vi "Teleop.vi"(10 "Match Info":T1={"Autonomous Elapsed Seconds"=0.0, "TeleOp Elapsed Seconds"=0.0, "Disabled Elapsed Seconds"=0.0, "Visited Autonomous"=FALSE, "Visited TeleOp"=FALSE, "Visited Disabled"=FALSE, "Autonomous Settings"={"Autonomous Style"=enum."Independent", "VI Refnum"=refnum}}, 11 "Call Context":T2) -> ()   [LabVIEW 2019]
doc: "This VI is called for each TeleOp packet received from the DS where the robot is not disabled. It is often used to read from the joysticks and update I/O or to update setpoints for timed control loops. It should complete and return within 20 milliseconds or it may miss DS packets."
uses:
  <vilib>/Rock Robotics/WPI/DriverStation/WPI_DriverStationDerivedRobotMode.ctl
  <vilib>/Rock Robotics/WPI/DriverStation/WPI_DriverStationMatch Info.ctl
  <vilib>/Rock Robotics/WPI/ThirdParty/REV Robotics/SPARK MAX/Typedef/Spark MAX Idle Mode.ctl
  Robot Global Data.vi
panel:
  # "Click here to set max"
  # "Click here to set min"
  # "Click here to set max"
  # "Click here to set min"
  # "Click here to set max"
  # "Click here to set min"
  # "Click here to set max"
  # "Click here to set min"
  # "Click here to set max"
  # "Click here to set min"
  # "Click here to set max"
  # "Click here to set min"
  # "Click here to set max"
  # "Click here to set min"
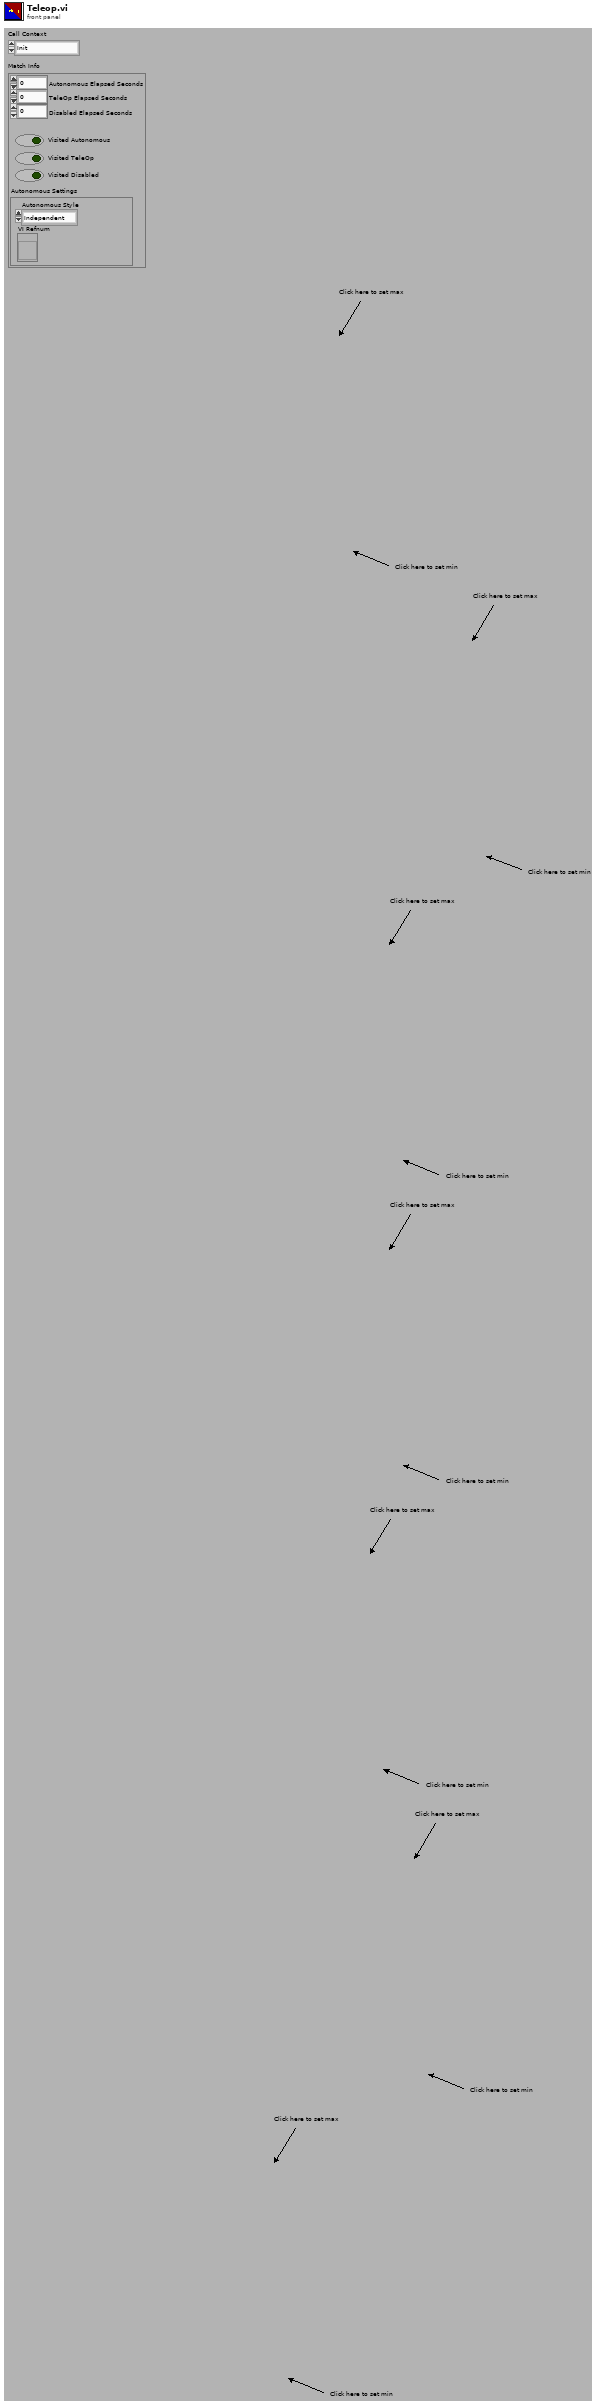
[diagram p1: front panel]
types:
  T1 = typedef "WPI_DriverStationMatch Info.ctl" = cluster{"Autonomous Elapsed Seconds":dbl, "TeleOp Elapsed Seconds":dbl, "Disabled Elapsed Seconds":dbl, "Visited Autonomous":bool, "Visited TeleOp":bool, "Visited Disabled":bool, "Autonomous Settings":cluster{"Autonomous Style":enum16{"Iterative", "Independent"}, "VI Refnum":refnum<vi>}}
  T2 = typedef "WPI_DriverStationDerivedRobotMode.ctl" = enum16{"Init", "Execute", "Stop"}
  T3 = typedef "WPI_MotorControlDeviceRef.ctl" = cluster{"DeviceStatus":errorcluster, "Type":T4, "PWM":cluster{"PWM Channel":T5, "DeadBand":T6}, "CAN":cluster{"Device Number":u8, "SetOutput VI Ref":variant, "GetOutput VI Ref":variant, "Enable VI Ref":variant, "Disable VI Ref":variant, "Data":variant}, "Invert":bool, "DIO PWM":cluster{"PWM \"Enable\" Channel":T5, "DIOChannel":T7, "PWM Rate":dbl}}
  T4 = typedef "WPI_MotorControlType.ctl" = enum16{"PWM", "CAN", "DIO PWM"}
  T5 = typedef "FPGA_DIOPWMChannel.ctl" = enum8{"PWM 0", "PWM 1", "PWM 2", "PWM 3", "PWM 4", "PWM 5", "PWM 6", "PWM 7", "PWM 8", "PWM 9", "PWM MXP 0", "PWM MXP 1", "PWM MXP 2", "PWM MXP 3", "PWM MXP 4", "PWM MXP 5", "PWM MXP 6", "PWM MXP 7", "PWM MXP 8", "PWM MXP 9", "Invalid"}
  T6 = typedef "WPI_PWMDeadband.ctl" = cluster{"Name":string, "maxPositivePwm":i32, "minPositivePwm":i32, "centerPwm":i32, "maxNegativePwm":i32, "minNegativePwm":i32, "angularRange":u16}
  T7 = typedef "FPGA_DIOChannel.ctl" = enum8{"DIO 0", "DIO 1", "DIO 2", "DIO 3", "DIO 4", "DIO 5", "DIO 6", "DIO 7", "DIO 8", "DIO 9", "DIO MXP 0", "DIO MXP 1", "DIO MXP 2", "DIO MXP 3", "DIO MXP 4", "DIO MXP 5", "DIO MXP 6", "DIO MXP 7", "DIO MXP 8", "DIO MXP 9", "DIO MXP 10", "DIO MXP 11", "DIO MXP 12", "DIO MXP 13", "DIO MXP 14", "DIO MXP 15", "SPI Port CS1", "SPI Port CS2", "SPI Port CS3", "SPI Port MISO", "SPI Port MOSI", "Invalid"}
  T8 = typedef "WPI_ServoDeviceRef.ctl" = cluster{"DeviceStatus":errorcluster, "PWM Channel":T5, "DeadBand":T6}
  T9 = typedef "Spark MAX Idle Mode.ctl" = enum16{"Coast", "Brake"}
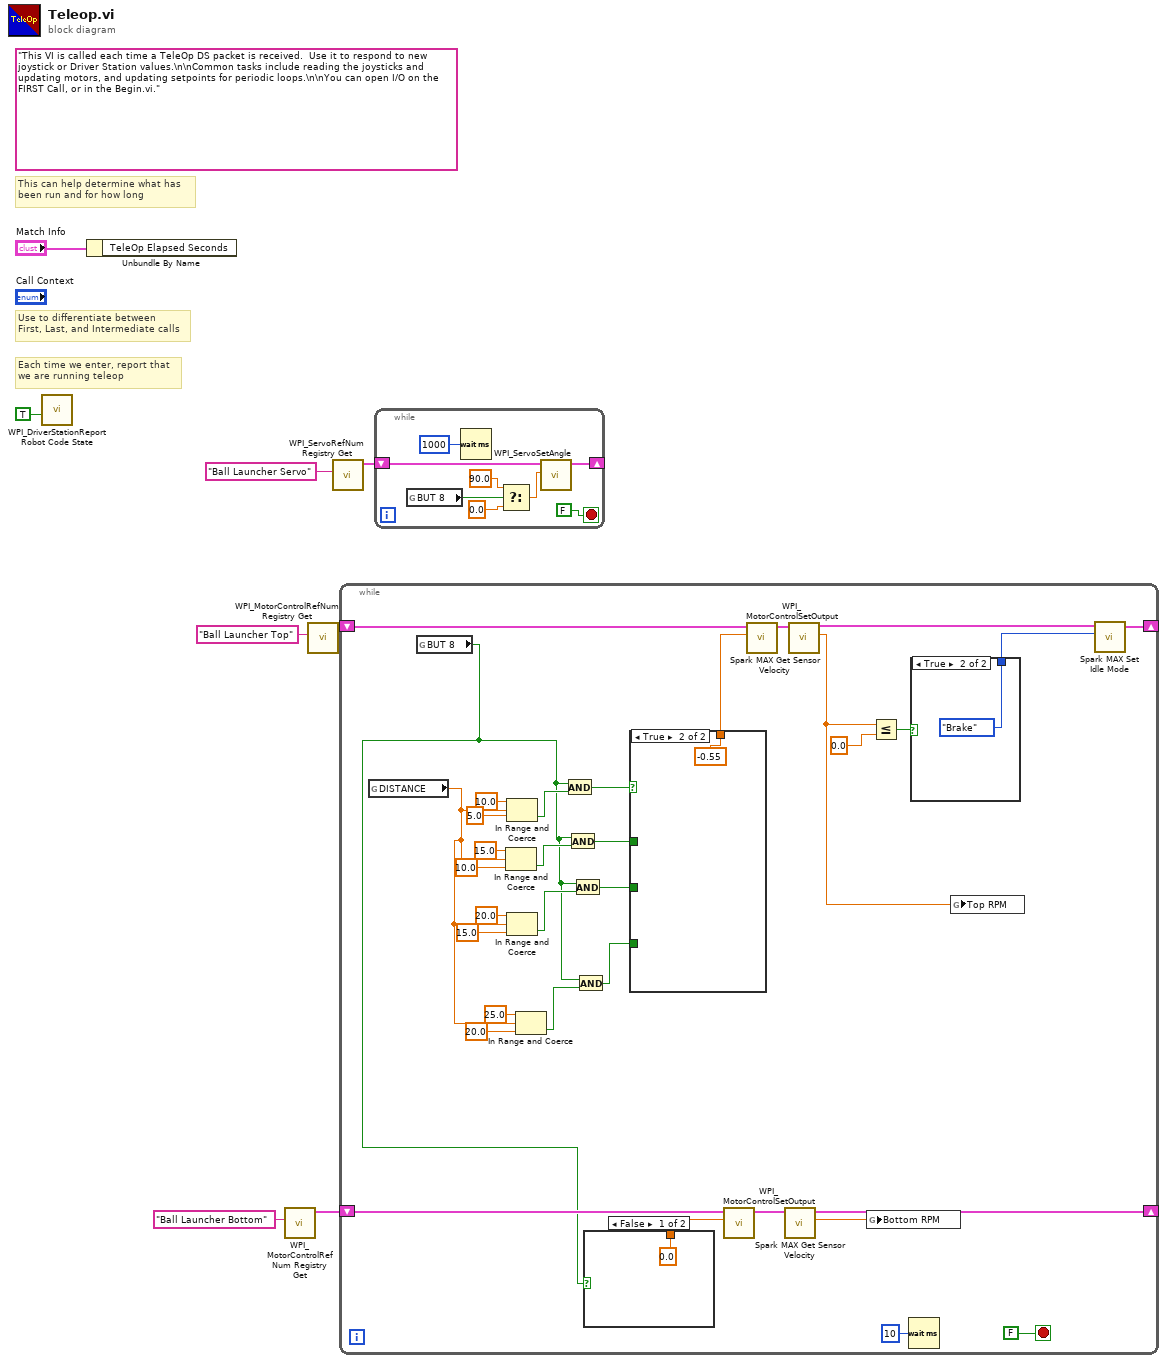
[diagram p0: block diagram]
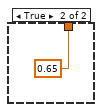
[diagram p2: hidden frame]
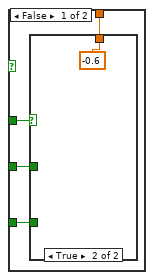
[diagram p3: hidden frame]
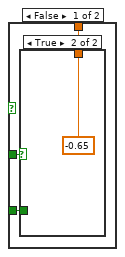
[diagram p4: hidden frame]
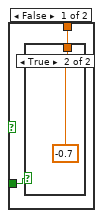
[diagram p5: hidden frame]
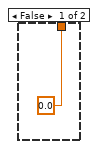
[diagram p6: hidden frame]
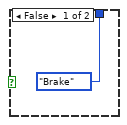
[diagram p7: hidden frame]
diagram:
  (unwired) "This VI is called each time a TeleOp DS packet is received.  Use it to respond to new joystick or Driver Station values.\n\nCommon tasks include reading the joysticks and updating motors, and updating setpoints for periodic loops.\n\nYou can open I/O on the FIRST Call, or in the Begin.vi."
  # "Each time we enter, report that\nwe are running teleop"
  # "Use to differentiate between\nFirst, Last, and Intermediate calls"
  # "This can help determine what has\nbeen run and for how long"
  n1 = call <vilib>:"WPI_DriverStationReport Robot Code State.vi"("TeleOp"=TRUE ("Autonomous")) -> ()  [unwired: 10 in, 1 out]
  n2 = Unbundle By Name("Match Info") -> ()  [unwired: 1 out]
  n3 = call <vilib>:"WPI_MotorControlRefNum Registry Get.vi"("refnum name"="Ball Launcher Bottom") -> ("MotorControlDevRef"=w1:T3)  [unwired: 9 in, 1 out]
  n4 = call <vilib>:"WPI_MotorControlRefNum Registry Get.vi"("refnum name"="Ball Launcher Top") -> ("MotorControlDevRef"=w4:T3)  [unwired: 9 in, 1 out]
  n5 = call <vilib>:"WPI_ServoRefNum Registry Get.vi"("refnum name"="Ball Launcher Servo") -> ("ServoDeviceRef"=w6:T8)  [unwired: 9 in, 1 out]
  n6 = while {
    shift-right: [w37] -> _
    shift-left: w4 -> [w41]
    shift-right: [w32] -> _
    shift-left: w1 -> [w34]
    stop <- FALSE stop-if-true
    n7 = global read "Robot Global Data.vi" "DISTANCE"() -> (w15:dbl)
    n8 = global read "Robot Global Data.vi" "BUT 8"() -> (w10:bool)
    n9 = In Range and Coerce(upper limit=15.0, x=w15, lower limit=10.0) -> (In Range?=w22:bool)  [unwired: 1 out]
    n10 = In Range and Coerce(upper limit=10.0, x=w15, lower limit=5.0) -> (In Range?=w27:bool)  [unwired: 1 out]
    n11 = In Range and Coerce(upper limit=20.0, x=w15, lower limit=15.0) -> (In Range?=w19:bool)  [unwired: 1 out]
    n12 = In Range and Coerce(upper limit=25.0, x=w15, lower limit=20.0) -> (In Range?=w9:bool)  [unwired: 1 out]
    n13 = And(x=w10, y=w27) -> (x .and. y?=w28:bool)
    n14 = And(x=w10, y=w22) -> (x .and. y?=w21:bool)
    n15 = And(x=w10, y=w19) -> (x .and. y?=w20:bool)
    n16 = And(x=w10, y=w9) -> (x .and. y?=w16:bool)
    n17 = case shown="False" w10 {
      tunnel: [0.0 ("Output") 0.65 ("Output")] -> w11
      frame False {
      }
      frame True {
      }
    }
    n18 = case shown="True" w28 {
      tunnel: w21 -> [w48 _]
      tunnel: w20 -> [w47 _]
      tunnel: w16 -> [w46 _]
      tunnel: [w45 -0.55 ("Output")] -> w12
      frame False {
        n19 = case shown="True" w48 {
          tunnel: w47 -> [w51 _]
          tunnel: w46 -> [w50 _]
          tunnel: [w49 -0.6 ("Output")] -> w45
          frame False {
            n20 = case shown="True" w51 {
              tunnel: w50 -> [w53 _]
              tunnel: [w52 -0.65 ("Output")] -> w49
              frame False {
                n21 = case shown="True" w53 {
                  tunnel: [0.0 ("Output") -0.7 ("Output")] -> w52
                  frame False {
                  }
                  frame True {
                  }
                }
              }
              frame True {
              }
            }
          }
          frame True {
          }
        }
      }
      frame True {
      }
    }
    n22 = call <vilib>:"WPI_MotorControlSetOutput.vi"("Output"=w11, "MotorControlDevRef"=w34) -> ("MotorControlDevRef"=w33:T3)  [unwired: 7 in, 2 out]
    n23 = call <vilib>:"WPI_MotorControlSetOutput.vi"("Output"=w12, "MotorControlDevRef"=w41) -> ("MotorControlDevRef"=w42:T3)  [unwired: 7 in, 2 out]
    n24 = call <vilib>:"Spark MAX Get Sensor Velocity.vi"("MotorControlDevRef in"=w33) -> ("Sensor Velocity"=w30:dbl, "MotorControlDevRef out"=w32:T3)  [unwired: 7 in, 2 out]
    n25 = call <vilib>:"Spark MAX Get Sensor Velocity.vi"("MotorControlDevRef in"=w42) -> ("Sensor Velocity"=w31:dbl, "MotorControlDevRef out"=w36:T3)  [unwired: 7 in, 2 out]
    n26 = global write "Robot Global Data.vi" "Bottom RPM"(w30) -> ()
    n27 = Less Or Equal?(x=w31, y=0.0) -> (x <= y?=w29:bool)
    n28 = Wait (ms)(milliseconds to wait=u32 10) -> ()  [unwired: 1 out]
    n29 = case shown="True" w29 {
      tunnel: [Spark_MAX_Idle_Mode."Brake" ("Idle Mode") Spark_MAX_Idle_Mode."Brake" ("Idle Mode")] -> w35
      frame False {
      }
      frame True {
      }
    }
    n30 = global write "Robot Global Data.vi" "Top RPM"(w31) -> ()
    n31 = call <vilib>:"Spark MAX Set Idle Mode.vi"("Idle Mode"=w35, "MotorControlDeviceRef in"=w36) -> ("MotorControlDeviceRef out"=w37:T3)  [unwired: 8 in, 1 out]
  }
  n32 = while {
    shift-right: [w64] -> _
    shift-left: w6 -> [w63]
    stop <- FALSE stop-if-true
    n33 = global read "Robot Global Data.vi" "BUT 8"() -> (w61:bool)
    n34 = Wait (ms)(milliseconds to wait=u32 1000) -> ()  [unwired: 1 out]
    n35 = Select(t=90.0, s=w61, f=0.0) -> (s? t:f=w62:dbl)
    n36 = call <vilib>:"WPI_ServoSetAngle.vi"("Angle"=w62, "ServoDeviceRef"=w63) -> ("ServoDeviceRef"=w64:T8)  [unwired: 8 in, 1 out]
  }
